vi "set_mag_inputs.vi"(8 "error in (no error)":errorcluster, 10 "mag inputs":T1, 11 "magnetometer in":refnum<class "magnetometer.lvclass">) -> (0 "error out":errorcluster, 3 "magnetometer out":refnum<class "magnetometer.lvclass">)   [LabVIEW 2015, in "magnetometer.lvclass"]
uses:
  magnetometer.lvclass
  magnetometer.lvclass/magnetometer.ctl
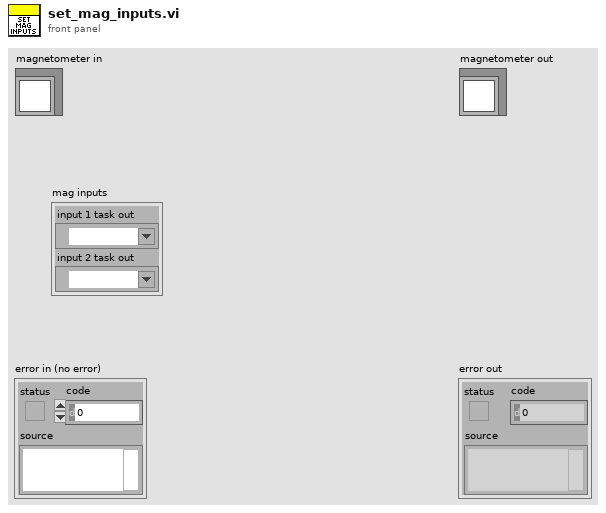
[diagram p1: front panel]
types:
  T1 = cluster{"input 1 task out":refnum<k21>, "input 2 task out":refnum<k21>}
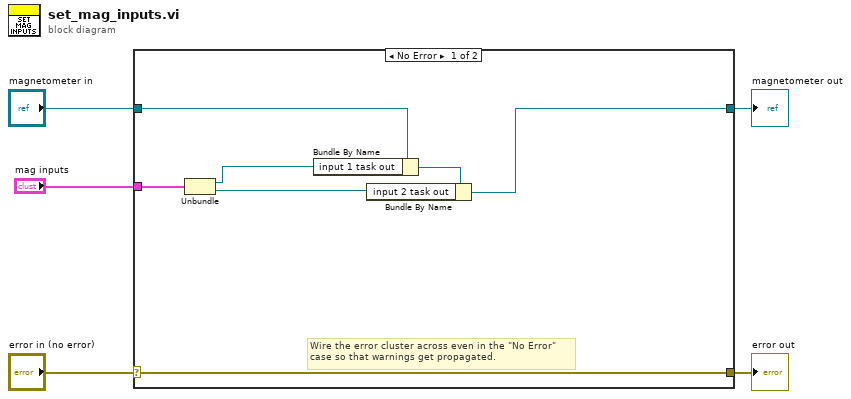
[diagram p0: block diagram]
diagram:
  n1 = case shown="No Error" "error in (no error)" {
    selector: "error in (no error)" -> [w12 w14]
    tunnel: [w12 w14] -> w4
    tunnel: [w9 w13] -> w2
    tunnel: "magnetometer in" -> [w11 w13]
    tunnel: "mag inputs" -> [w8 _]
    frame No Error {
      # "Wire the error cluster across even in the \"No Error\"\ncase so that warnings get propagated."
      n2 = Unbundle(w8) -> ("input 1 task out"=w7:refnum<k21>, "input 2 task out"=w6:refnum<k21>)
      n3 = Bundle By Name(cluster=w11, "input 1 task out"=w7) -> (w10:refnum<class "magnetometer.lvclass">)
      n4 = Bundle By Name(cluster=w10, "input 2 task out"=w6) -> (w9:refnum<class "magnetometer.lvclass">)
    }
    frame Error {
    }
  }
  "error out" <- w4
  "magnetometer out" <- w2
